vi "Auto_Routine_StraightThreePieceLeftNoteTRAJ.vi"(8 "error in (no error)":errorcluster) -> (0 "error out":errorcluster)   [LabVIEW 2023]
uses:
  Trajectory/TrajectoryGlobals.vi
  <vilib>/Rock Robotics/WPI/ThirdParty/JAS_Junk/TrajLib/Trajectory_Library.lvlib
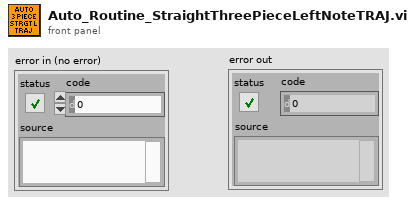
[diagram p1: front panel]
types:
  T1 = typedef "Trajectory_Library.lvlib/TRAJECTORY.ctl" = cluster{"TotalTImeSecs":dbl, "States":T2[]}
  T2 = typedef "Trajectory_Library.lvlib/TRAJ_STATE.ctl" = cluster{"TimeSeconds":dbl, "Velocity":dbl, "Acceleration":dbl, "POSE":T3, "Curvature":dbl}
  T3 = typedef "Trajectory_Library.lvlib/POSE2D.ctl" = cluster{"TRANSLATION":T4, "ROTATION":T5}
  T4 = typedef "Trajectory_Library.lvlib/TRANSLATION2D.ctl" = cluster{"X":dbl, "Y":dbl}
  T5 = typedef "Trajectory_Library.lvlib/ROTATION2D.ctl" = cluster{"VALUE":dbl, "COS":dbl, "SIN":dbl}
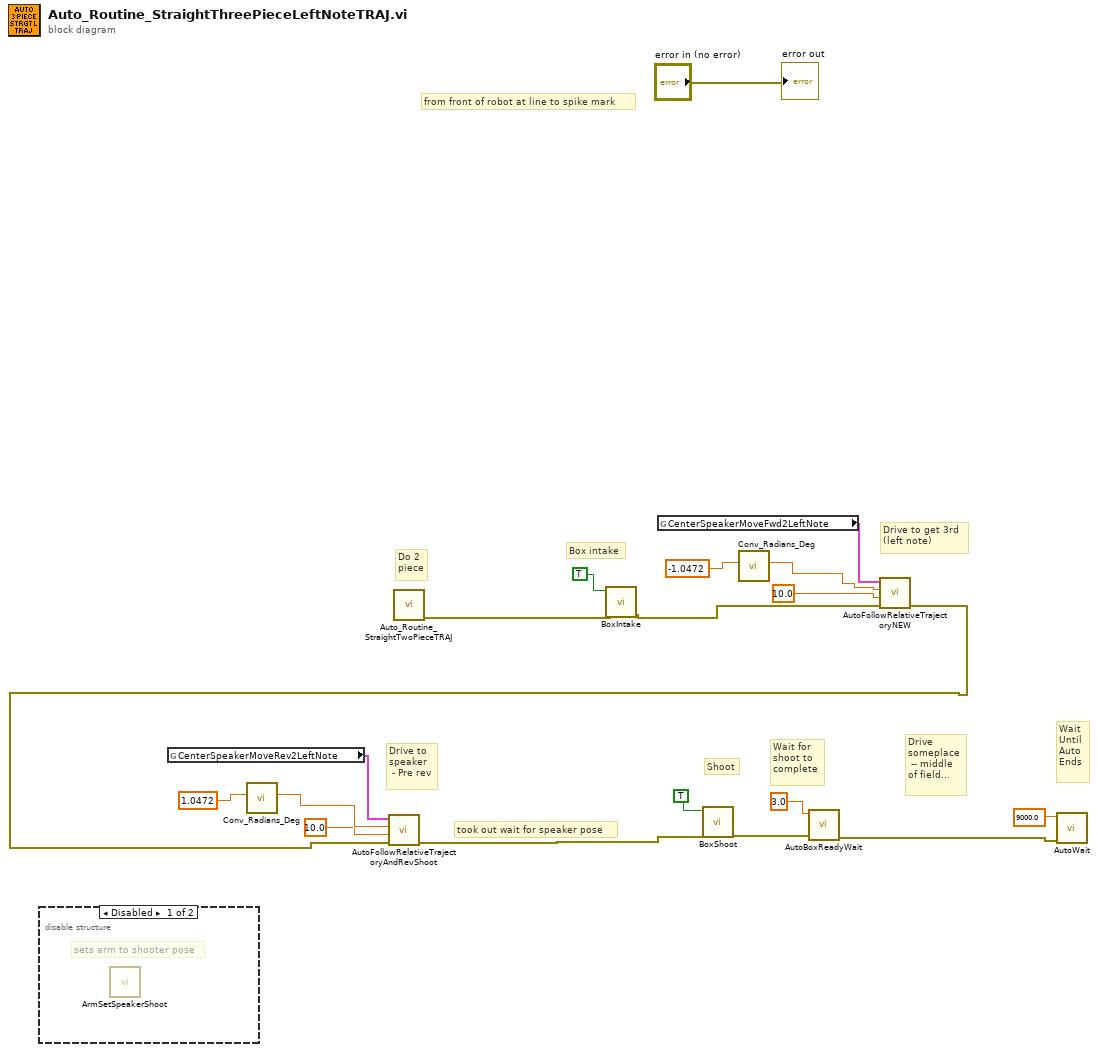
[diagram p0: block diagram]
diagram:
  # "took out wait for speaker pose"
  # "Drive to get 3rd \n(left note)"
  # "Do 2 \npiece"
  # "Drive\nsomeplace\n -- middle\nof field..."
  # "Box intake"
  # "Wait for\nshoot to\ncomplete"
  # "Shoot"
  # "Drive to\nspeaker\n - Pre rev"
  # "Wait\nUntil\nAuto \nEnds"
  # "from front of robot at line to spike mark"
  n1 = disable-structure shown="Disabled" {
    frame Disabled {
      # "sets arm to shooter pose"
      n2 = call "ArmSetSpeakerShoot.vi"() -> ()  [unwired: 11 in, 1 out]
    }
    frame Enabled {
    }
  }
  n3 = global read "TrajectoryGlobals.vi" "CenterSpeakerMoveRev2LeftNote"() -> (w11:T1)
  n4 = call <vilib>:"Conv_Radians_Deg.vi"("Radians"=1.0472) -> ("Degrees"=w9:dbl)  [unwired: 10 in]
  n5 = call "Auto_Routine_StraightTwoPieceTRAJ.vi"() -> ("error out"=w5:errorcluster)  [unwired: 11 in]
  n6 = call "BoxIntake.vi"("error in (no error)"=w5, "Box intake"=TRUE) -> ("error out"=w6:errorcluster)  [unwired: 9 in]
  n7 = global read "TrajectoryGlobals.vi" "CenterSpeakerMoveFwd2LeftNote"() -> (w17:T1)
  n8 = call <vilib>:"Conv_Radians_Deg.vi"("Radians"=-1.0472) -> ("Degrees"=w3:dbl)  [unwired: 10 in]
  n9 = call "AutoFollowRelativeTrajectoryNEW.vi"("error in (no error)"=w6, "TimeOut (s)"=10.0, "End Orientation"=w3, "Trajectory"=w17) -> ("error out"=w1:errorcluster)  [unwired: 7 in]
  n10 = call "AutoFollowRelativeTrajectoryAndRevShoot.vi"("error in (no error)"=w1, "TimeOut (s)"=10.0, "End Orientation"=w9, "Trajectory"=w11) -> ("error out"=w2:errorcluster)  [unwired: 7 in]
  n11 = call "BoxShoot.vi"("error in (no error)"=w2, "Box shoot"=TRUE) -> ("error out"=w14:errorcluster)  [unwired: 9 in]
  n12 = call "AutoBoxReadyWait.vi"("error in (no error)"=w14, "TimeOut (s)"=3.0) -> ("error out"=w12:errorcluster)  [unwired: 9 in]
  n13 = call "AutoWait.vi"("error in (no error)"=w12, "TimeOut (s)"=9000.0) -> ()  [unwired: 9 in, 1 out]
  "error out" <- "error in (no error)"
